vi "write.vi"(8 "error in (no error)":errorcluster, 10 "writeString":string, 11 "SerialSimulator in":refnum<class "SerialSimulator.lvclass">) -> (0 "error out":errorcluster, 3 "SerialSimulator out":refnum<class "SerialSimulator.lvclass">)   [LabVIEW 2015, in "SerialProtocols.lvlib" / "SerialSimulator.lvclass"]
uses:
  <userlib>/Common/SerialProtocols/SerialProtocol/SerialSimulator/SerialSimulator.lvclass
  <userlib>/Common/SerialProtocols/SerialProtocol/SerialSimulator/SerialSimulator.lvclass/SerialSimulator.ctl
  <userlib>/Common/Simulators/SimulateSerialData/SimulateSerialData.lvclass
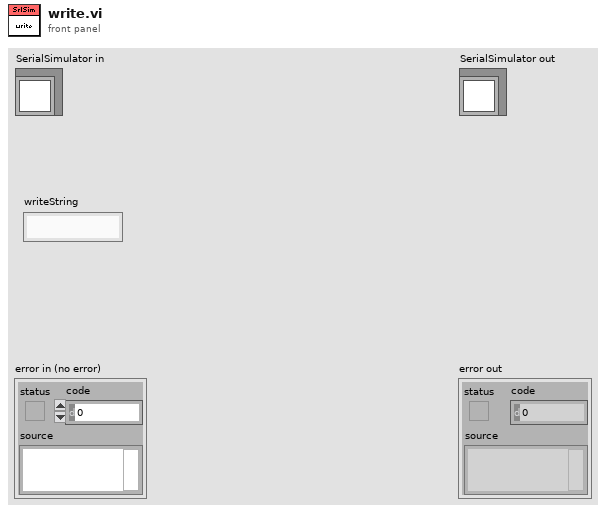
[diagram p1: front panel]
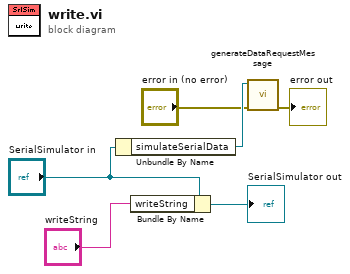
[diagram p0: block diagram]
diagram:
  n1 = Unbundle By Name("SerialSimulator in") -> ("simulateSerialData"=w6:refnum<class "SimulateSerialData.lvclass">)
  n2 = Bundle By Name(cluster="SerialSimulator in", "writeString"="writeString") -> (→"SerialSimulator out":refnum<class "SerialSimulator.lvclass">)
  n3 = call-dynamic "generateDataRequestMessage.vi"("error in (no error)"="error in (no error)", "SimulateSerialData in"=w6) -> ("error out"=→"error out":errorcluster)  [unwired: 8 in, 1 out]
